vi "Calculate Angles.vi"(5 "Robot Orientation":T1, 6 "Right Angle In":dbl, 7 "Left Angle In":dbl) -> (0 "Rear Right Steer Out":dbl, 1 "Rear Left Pot Out":dbl, 2 "Front Right Pot Out":dbl, 3 "Front Left Pot Out":dbl)   [LabVIEW 2012]
uses:
  Controls/Robot Orientation.ctl
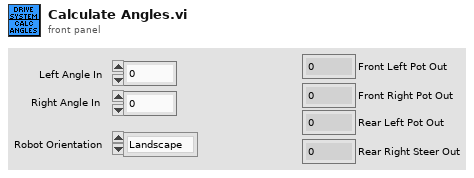
[diagram p1: front panel]
types:
  T1 = typedef "Robot Orientation.ctl" = enum16{"Landscape", "Portrait"}
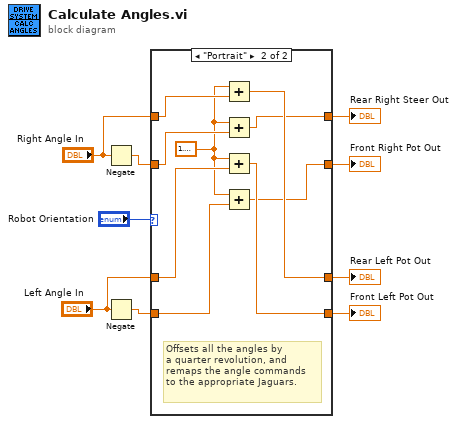
[diagram p0: block diagram]
diagram:
  n1 = Negate(x="Right Angle In") -> (-x=w8:dbl)
  n2 = Negate(x="Left Angle In") -> (-x=w5:dbl)
  n3 = case shown="\"Portrait\"" "Robot Orientation" {
    tunnel: "Right Angle In" -> [w13 w22]
    tunnel: [w13 w19] -> w9
    tunnel: w8 -> [w12 w20]
    tunnel: [w12 w14] -> w7
    tunnel: "Left Angle In" -> [w11 w18]
    tunnel: [w11 w21] -> w6
    tunnel: w5 -> [w10 w15]
    tunnel: [w10 w17] -> w3
    frame "Landscape", Default {
    }
    frame "Portrait" {
      w16 = 1.5707963267948966
      # "Offsets all the angles by\na quarter revolution, and\nremaps the angle commands\nto the appropriate Jaguars."
      n4 = Add(x=w16, y=w22) -> (x+y=w21:dbl)
      n5 = Add(x=w16, y=w20) -> (x+y=w19:dbl)
      n6 = Add(x=w16, y=w18) -> (x+y=w17:dbl)
      n7 = Add(x=w16, y=w15) -> (x+y=w14:dbl)
    }
  }
  "Front Left Pot Out" <- w3
  "Front Right Pot Out" <- w7
  "Rear Left Pot Out" <- w6
  "Rear Right Steer Out" <- w9
